vi "Test Helper Loop Errors sent to Error Handler.vi"(8 "error in (no error)":errorcluster, 11 "Helper Loop Test In":refnum<class "Helper Loop Test.lvclass">) -> (0 "error out":errorcluster, 3 "Helper Loop Test Out":refnum<class "Helper Loop Test.lvclass">)   [LabVIEW 2020, in "Helper Loop Test.lvclass"]
uses:
  Helper Loop Test.lvclass
  C:/Program Files (x86)/National Instruments/LabVIEW 2020/vi.lib/Astemes/LUnit/Test Case.lvclass
  source/Framework Test Suite/Mock Process/Mock Process.lvclass
  C:/Git/astemes-triarc-framework/source/Framework/Process/Process.lvclass
  source/Framework Test Suite/Mock Error Handler/Mock Error Handler.lvclass
  C:/Git/astemes-triarc-framework/source/Framework/Error Handler Interface/Error Handler Interface.lvclass
  source/Framework/Process/Process.lvclass/Process.ctl
  <vilib>/Astemes/LUnit/Test Case.lvclass/Test Case.ctl
  <vilib>/Astemes/LUnit/LUnit Assertion Result.lvclass/LUnit Assertion Result.ctl
  <vilib>/Astemes/LUnit/LUnit Test Case Result.lvclass/LUnit Test Case Result.ctl
  <vilib>/Astemes/LUnit/LUnit Method Result.lvclass/LUnit Method Result.ctl
  source/Framework/Process/Protected/Messaging/Enqueue Message.vi
  source/Framework/Process/Public/Lifecycle/Get Lifecycle State.vi
  <vilib>/Astemes/LUnit/Palette/Pass If Equal.vi/cbf50e99-f124-4847-863a-8e9794d3dede.vi
  source/Framework/Process/Private/SubVIs/Wait for finish.vi
  source/Framework/Process/Private/SubVIs/Set Lifecycle State.vi
  source/Framework/Process/Private/SubVIs/Handle Debug Data.vi
  <vilib>/Utility/error.llb/Clear Errors.vi
  <vilib>/Astemes/LUnit/Palette/Pass.vi
  <vilib>/Astemes/LUnit/Palette/Fail.vi
  <vilib>/Astemes/LUnit/Compare Variants.vi
  <vilib>/Astemes/LUnit/Describe Comparison.vi
  <vilib>/Astemes/LUnit/Set Assertion Type.vi
  source/Framework/Logging/Log Debug.vi
  <vilib>/AdvancedString/1D String Array to Delimited String.vi
  <vilib>/Utility/High Resolution Relative Seconds.vi
  <vilib>/Astemes/LUnit/Add test result.vi
  <vilib>/Astemes/LUnit/LUnit Write Passed.vi
  <vilib>/Astemes/LUnit/LUnit Write Message.vi
  <vilib>/Astemes/LUnit/LUnit Write Description.vi
  <vilib>/Astemes/LUnit/Variant to string.vi
  <vilib>/Astemes/LUnit/LUnit Write Assertion Type.vi
  <vilib>/Astemes/LUnit/LUnit Record Assertion Result.vi
  <vilib>/Astemes/LUnit/LUnit Aggregate Assertion Results.vi
  <vilib>/Astemes/LUnit/Assertion Result/LUnit Read Status.vi
  <vilib>/Astemes/LUnit/LUnit Read Message.vi
  <vilib>/Astemes/LUnit/LUnit Read Description.vi
  <vilib>/Astemes/LUnit/Method Result/LUnit Merge Status.vi
  <vilib>/Astemes/LUnit/LUnit Concatenate result strings.vi
  <vilib>/Utility/error.llb/Error Cluster From Error Code.vi
  source/Framework/Process/Public/Read Name.vi
  <vilib>/Utility/Data Type/Get Type Information.vi
  <vilib>/Utility/LVClass/Get LV Class Name.vi
  <vilib>/Astemes/LUnit/LUnit Assertion Result.lvclass
  source/Framework/Process/Process.lvclass
  Helper Loop Test.lvclass/Helper Loop Test.ctl
  <vilib>/Astemes/LUnit/Test Case.lvclass
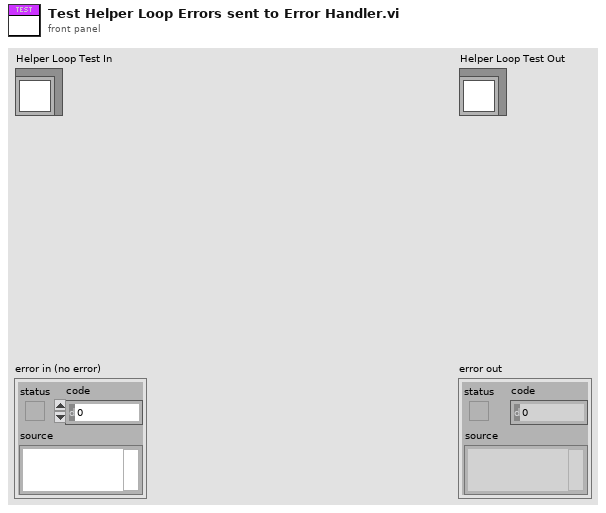
[diagram p1: front panel]
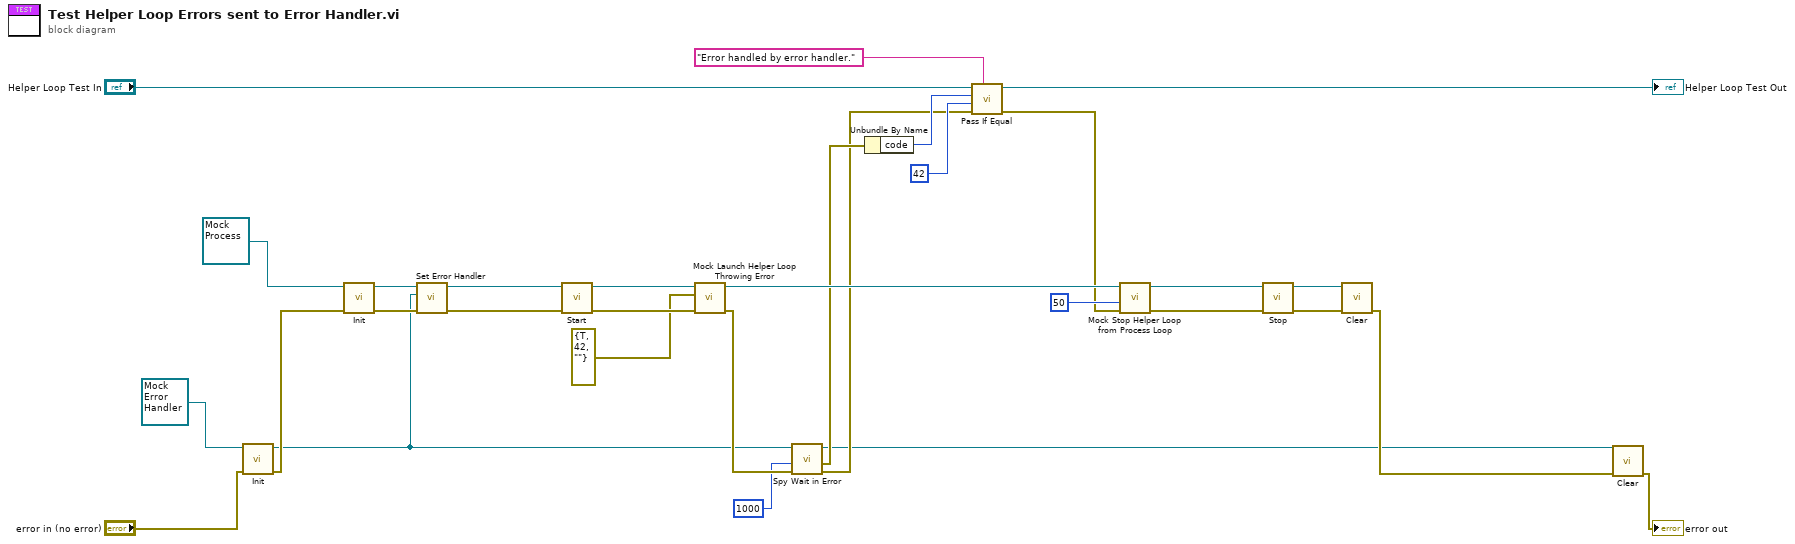
[diagram p0: block diagram]
diagram:
  n1 = call-dynamic "Init.vi"("error in (no error)"="error in (no error)", "Mock Error Handler In"=refnum<class "Mock Error Handler.lvclass"> refnum) -> ("error out"=w4:errorcluster, "Mock Error Handler Out"=w3:refnum<class "Mock Error Handler.lvclass">)  [unwired: 8 in]
  n2 = call-dynamic "Init.vi"("error in (no error)"=w4, "Mock Process In"=refnum<class "Mock Process.lvclass"> refnum) -> ("error out"=w19:errorcluster, "Mock Process Out"=w31:refnum<class "Mock Process.lvclass">)  [unwired: 8 in]
  n3 = call "Set Error Handler.vi"("error in (no error)"=w19, "Error Handler"=w3, "Process In"=w31) -> ("error out"=w18:errorcluster, "Process Out"=w20:refnum<class "Mock Process.lvclass">)  [unwired: 7 in]
  n4 = call "Start.vi"("error in (no error)"=w18, "Process In"=w20) -> ("error out"=w29:errorcluster, "Process Out"=w30:refnum<class "Mock Process.lvclass">)  [unwired: 7 in, 1 out]
  n5 = call "Mock Launch Helper Loop Throwing Error.vi"("error in (no error)"=w29, "Error message"=errorcluster {"status"=TRUE, "code"=42, "source"=""}, "Mock Process in"=w30) -> ("error out"=w15:errorcluster, "Mock Process out"=w28:refnum<class "Mock Process.lvclass">)  [unwired: 7 in]
  n6 = call "Spy Wait in Error.vi"("error in (no error)"=w15, "timeout in ms (-1)"=1000, "Mock Error Handler In"=w3) -> ("error out"=w5:errorcluster, "Errors"=w9:errorcluster, "Mock Error Handler Out"=w2:refnum<class "Mock Error Handler.lvclass">)  [unwired: 4 in, 2 out]
  n7 = Unbundle By Name(w9) -> ("code"=w8:i32)
  n8 = call <vilib>:"Pass If Equal.vi"("Description"="Error handled by error handler.", "error in (no error)"=w5, "Actual"=42 ("code"), "Expected"=w8, "LUnit Test Case In"="Helper Loop Test In") -> ("error out"=w11:errorcluster, "LUnit Test Case Out"=→"Helper Loop Test Out":refnum<class "Helper Loop Test.lvclass">)  [unwired: 5 in]
  n9 = call "Mock Stop Helper Loop from Process Loop.vi"("error in (no error)"=w11, "timeout in ms (-1)"=50, "Mock Process in"=w28) -> ("error out"=w26:errorcluster, "Mock Process out"=w27:refnum<class "Mock Process.lvclass">)  [unwired: 6 in, 1 out]
  n10 = call "Stop.vi"("error in (no error)"=w26, "Process In"=w27) -> ("error out"=w25:errorcluster, "Process Out"=w1:refnum<class "Mock Process.lvclass">)  [unwired: 7 in, 1 out]
  n11 = call-dynamic "Clear.vi"("error in (no error)"=w25, "Mock Process In"=w1) -> ("error out"=w24:errorcluster)  [unwired: 9 in]
  n12 = call-dynamic "Clear.vi"("error in (no error)"=w24, "Mock Process In"=w2) -> ("error out"=→"error out":errorcluster)  [unwired: 9 in]
